vi "TranslatePathSup.vi"(10 "Offset":T5, 11 "PathSupreme":T1) -> (3 "PathSupOut":T1)   [LabVIEW 2014]
uses:
  TypeDefs/PathSupreme.ctl
  PSup2SCAN/Sub/VelocityProfile.ctl
  PSup2SCAN/Sub/PathCut.ctl
  PSup2SCAN/Sub/Segment.ctl
  PSup2SCAN/Sub/Point.ctl
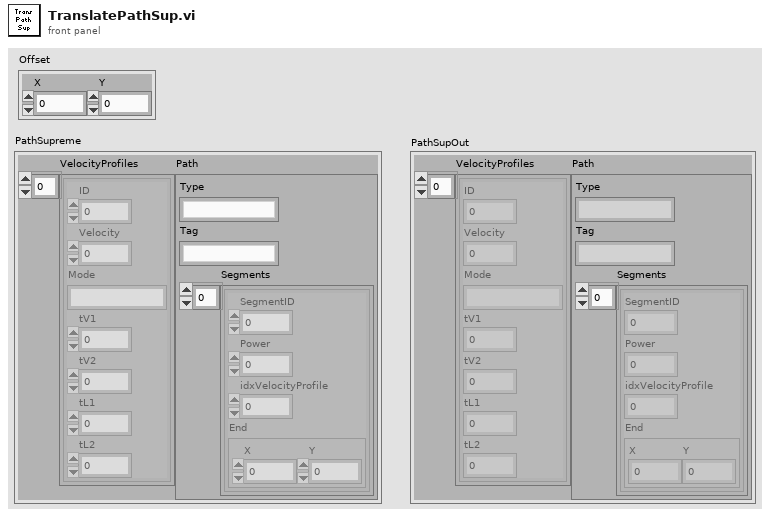
[diagram p1: front panel]
types:
  T1 = typedef "PathSupreme.ctl" = cluster{"VelocityProfiles":T2[], "Path":T3}
  T2 = typedef "VelocityProfile.ctl" = cluster{"ID":u32, "Velocity":dbl, "Mode":string, "tV1":u32, "tV2":u32, "tL1":u32, "tL2":u32}
  T3 = typedef "PathCut.ctl" = cluster{"Type":string, "Tag":string, "Segments":T4[]}
  T4 = typedef "Segment.ctl" = cluster{"SegmentID":u16, "Power":sgl, "idxVelocityProfile":u16, "End":cluster{"X":sgl, "Y":sgl}}
  T5 = typedef "Point.ctl" = cluster{"X":dbl, "Y":dbl}
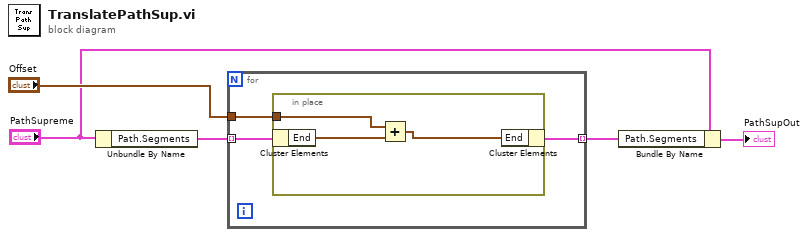
[diagram p0: block diagram]
diagram:
  n1 = Unbundle By Name("PathSupreme") -> ("Path.Segments"=w5:T4[])
  n2 = for {
    tunnel: w5 -> [w8] mode=indexing
    tunnel: "Offset" -> [w7]
    tunnel: [w6] -> w2 mode=indexing
    n3 = in-place {
      in-place-border: w7 -> [w10]
      n4 = in-place-cluster #1(w8) -> ("End"=w11:cluster{"X":sgl, "Y":sgl})
      n5 = Add(x=w10, y=w11) -> (x+y=w9:T5)
      n6 = in-place-cluster #1("End"=w9) -> (w6:T4)
    }
  }
  n7 = Bundle By Name(cluster="PathSupreme", "Path.Segments"=w2) -> (→"PathSupOut":T1)
